vi "DriveModuleReadEncoder.vi"(8 "error in":errorcluster, 11 "ModualNamePrefix":i32) -> (0 "error out":errorcluster, 2 "SWERVE_DRIVE_MODULE_POSITION":T1={"Distance"=0.0, "Angle"={"VALUE"=0.0, "COS"=1.0, "SIN"=0.0}, "P"=FALSE} {"Angle"."SIN" format="%13.4f"; "Angle"."COS" format="%13.4f"; "Angle"."VALUE" format="%13.4f"}, 3 "SWERVE_DRIVE_MODULE_STATE":T3={"Speed"=0.0, "Angle"={"VALUE"=0.0, "COS"=1.0, "SIN"=0.0}} {"Angle"."SIN" format="%13.4f"; "Angle"."COS" format="%13.4f"; "Angle"."VALUE" format="%13.4f"})   [LabVIEW 2023]
uses:
  <vilib>/Rock Robotics/WPI/ThirdParty/JAS_Junk/TrajLib/TypeDef/SWERVE_DRIVE_MODULE_STATE.ctl
  <vilib>/Rock Robotics/WPI/ThirdParty/JAS_Junk/TrajLib/TypeDef/ROTATION2D.ctl
  <vilib>/Rock Robotics/WPI/ThirdParty/JAS_Junk/TrajLib/TypeDef/SWERVE_DRIVE_MODULE_POSITION.ctl
  <vilib>/Rock Robotics/WPI/ThirdParty/JAS_Junk/TrajLib/Conv_Deg_Radians.vi
  <vilib>/Rock Robotics/WPI/ThirdParty/JAS_Junk/TrajLib/Rotation2d_CreateAngle.vi
  DriveGlobal.vi
  <vilib>/Rock Robotics/WPI/ThirdParty/Phoenix6/Phoenix6_Device_RefNumRegistryGet.vi
  <vilib>/Rock Robotics/WPI/MotorControl/WPI_MotorControlRefNum Registry Get.vi
  <vilib>/Rock Robotics/WPI/ThirdParty/REV Robotics/REVLib/SubVI/Public/SPARK Get Encoder Status Velocity.vi
  <vilib>/Rock Robotics/WPI/ThirdParty/REV Robotics/REVLib/SubVI/Public/SPARK Get Encoder Status Position.vi
  <vilib>/Rock Robotics/WPI/ThirdParty/Phoenix6/getters/GetCANcoder_AbsPosition.vi
  <vilib>/Rock Robotics/WPI/ThirdParty/JAS_Junk/TrajLib/Trajectory_Library.lvlib
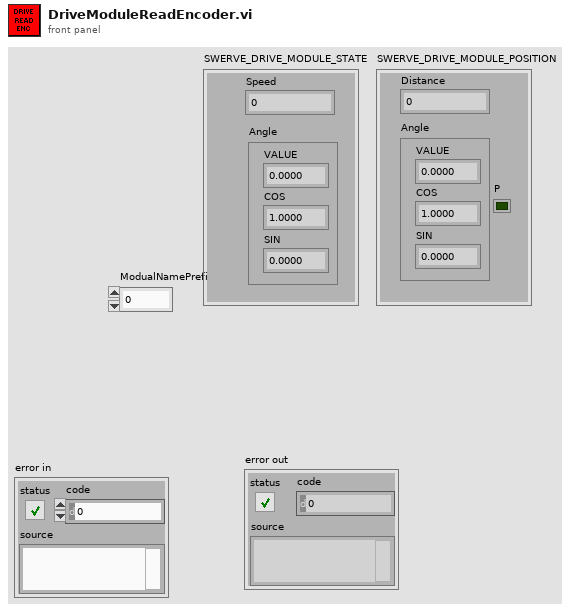
[diagram p1: front panel]
types:
  T1 = typedef "Trajectory_Library.lvlib/SWERVE_DRIVE_MODULE_POSITION.ctl" = cluster{"Distance":dbl, "Angle":T2, "P":bool}
  T2 = typedef "Trajectory_Library.lvlib/ROTATION2D.ctl" = cluster{"VALUE":dbl, "COS":dbl, "SIN":dbl}
  T3 = typedef "Trajectory_Library.lvlib/SWERVE_DRIVE_MODULE_STATE.ctl" = cluster{"Speed":dbl, "Angle":T2}
  T4 = typedef "WPI_MotorControlDeviceRef.ctl" = cluster{"DeviceStatus":errorcluster, "Type":T5, "PWM":cluster{"PWM Channel":T6, "DeadBand":T7}, "CAN":cluster{"Device Number":u8, "SetOutput VI Ref":variant, "GetOutput VI Ref":variant, "Enable VI Ref":variant, "Disable VI Ref":variant, "Data":variant}, "Invert":bool, "DIO PWM":cluster{"PWM \"Enable\" Channel":T6, "DIOChannel":T8, "PWM Rate":dbl}}
  T5 = typedef "WPI_MotorControlType.ctl" = enum16{"PWM", "CAN", "DIO PWM"}
  T6 = typedef "FPGA_DIOPWMChannel.ctl" = enum8{"PWM 0", "PWM 1", "PWM 2", "PWM 3", "PWM 4", "PWM 5", "PWM 6", "PWM 7", "PWM 8", "PWM 9", "PWM MXP 0", "PWM MXP 1", "PWM MXP 2", "PWM MXP 3", "PWM MXP 4", "PWM MXP 5", "PWM MXP 6", "PWM MXP 7", "PWM MXP 8", "PWM MXP 9", "Invalid"}
  T7 = typedef "WPI_PWMDeadband.ctl" = cluster{"Name":string, "maxPositivePwm":i32, "minPositivePwm":i32, "centerPwm":i32, "maxNegativePwm":i32, "minNegativePwm":i32, "angularRange":u16}
  T8 = typedef "FPGA_DIOChannel.ctl" = enum8{"DIO 0", "DIO 1", "DIO 2", "DIO 3", "DIO 4", "DIO 5", "DIO 6", "DIO 7", "DIO 8", "DIO 9", "DIO MXP 0", "DIO MXP 1", "DIO MXP 2", "DIO MXP 3", "DIO MXP 4", "DIO MXP 5", "DIO MXP 6", "DIO MXP 7", "DIO MXP 8", "DIO MXP 9", "DIO MXP 10", "DIO MXP 11", "DIO MXP 12", "DIO MXP 13", "DIO MXP 14", "DIO MXP 15", "SPI Port CS1", "SPI Port CS2", "SPI Port CS3", "SPI Port MISO", "SPI Port MOSI", "Invalid"}
  T9 = typedef "DeviceReference.ctl" = cluster{"CANbus Name":string, "Device Encoding":u32, "Device Name":string}
  T10 = cluster{"Value":dbl, "System Timestamp":dbl, "CANivore Timestamp":dbl, "ECU Timestamp":dbl}
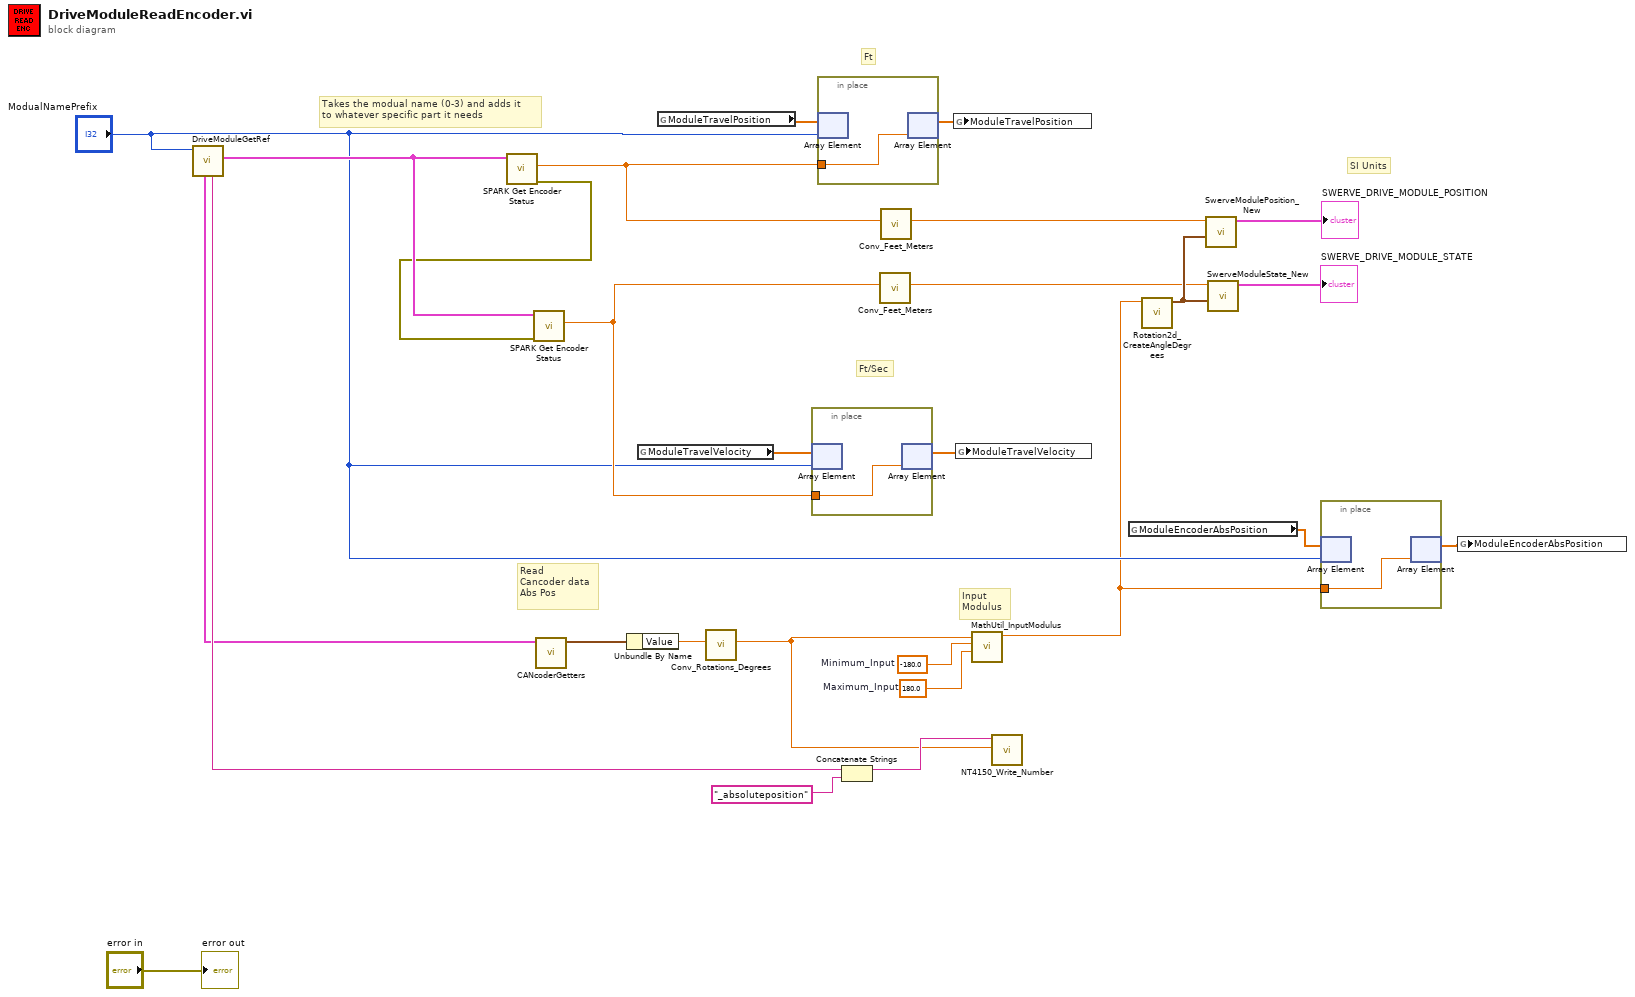
[diagram p0: block diagram]
diagram:
  w21 = -180.0  # Minimum_Input
  w20 = 180.0  # Maximum_Input
  # "SI Units"
  # "Ft/Sec"
  # "Ft"
  # "Read\nCancoder data\nAbs Pos"
  # "Input\nModulus"
  # "Takes the modual name (0-3) and adds it \nto whatever specific part it needs"
  n1 = call "DriveModuleGetRef.vi"("ModualNamePrefix"="ModualNamePrefix") -> ("TravMot"=w16:T4, "EncStr"=w17:string, "SpinAbsAngle"=w14:T9)  [unwired: 5 in, 3 out]
  n2 = call-poly <vilib>:"SPARK Get Encoder Status.vi"("MotorControlDevRef in"=w16) -> ("error out"=w15:errorcluster, "Sensor Position"=w9:dbl)  [unwired: 7 in, 2 out]
  n3 = call-poly <vilib>:"SPARK Get Encoder Status.vi"("error in (no error)"=w15, "MotorControlDevRef in"=w16) -> ("Sensor Velocity"=w5:dbl)  [unwired: 6 in, 3 out]
  n4 = call-poly <vilib>:"CANcoderGetters.vi"("DeviceReference"=w14) -> ("Output"=w13:T10)  [unwired: 9 in, 1 out]
  n5 = Unbundle By Name(w13) -> ("Value"=w12:dbl)
  n6 = global read "DriveGlobal.vi" "ModuleTravelVelocity"() -> (w7:dbl[])
  n7 = global read "DriveGlobal.vi" "ModuleTravelPosition"() -> (w10:dbl[])
  n8 = call <vilib>:"Conv_Rotations_Degrees.vi"("Rotations"=w12) -> ("Degrees"=w11:dbl)  [unwired: 10 in]
  n9 = in-place {
    in-place-border: w5 -> [w28]
    n10 = in-place-array #1(w7, "ModualNamePrefix") -> ()  [unwired: 1 out]
    n11 = in-place-array #1(w28) -> (w6:dbl[])  [unwired: 1 out]
  }
  n12 = in-place {
    in-place-border: w9 -> [w29]
    n13 = in-place-array #2(w10, "ModualNamePrefix") -> ()  [unwired: 1 out]
    n14 = in-place-array #2(w29) -> (w8:dbl[])  [unwired: 1 out]
  }
  n15 = Concatenate Strings(w17, "_absoluteposition" ("refnum name")) -> (w25:string)
  n16 = call <vilib>:"Conv_Feet_Meters.vi"("Feet"=w5) -> ("Meters"=w19:dbl)  [unwired: 10 in]
  n17 = call <vilib>:"Conv_Feet_Meters.vi"("Feet"=w9) -> ("Meters"=w18:dbl)  [unwired: 10 in]
  n18 = global write "DriveGlobal.vi" "ModuleTravelPosition"(w8) -> ()
  n19 = global write "DriveGlobal.vi" "ModuleTravelVelocity"(w6) -> ()
  n20 = call <vilib>:"MathUtil_InputModulus.vi"("Maximum_Input"=w20, "Minimum_Input"=w21, "Input"=w11) -> ("modulus"=w3:dbl)  [unwired: 8 in]
  n21 = call "NT4150_Write_Number.vi"("value"=w11, "name"=w25) -> ()  [unwired: 9 in, 1 out]
  n22 = global read "DriveGlobal.vi" "ModuleEncoderAbsPosition"() -> (w2:dbl[])
  n23 = call <vilib>:"Rotation2d_CreateAngleDegrees.vi"("Angle_Degrees"=w3) -> ("ROTATION"=w24:T2)  [unwired: 10 in]
  n24 = call <vilib>:"SwerveModulePosition_New.vi"("ROTATION"=w24, "Distance"=w18) -> ("SWERVE_DRIVE_MODULE_POSITION"=→"SWERVE_DRIVE_MODULE_POSITION":T1)  [unwired: 9 in]
  n25 = call <vilib>:"SwerveModuleState_New.vi"("ROTATION"=w24, "Speed"=w19) -> ("SWERVE_DRIVE_MODULE_STATE"=→"SWERVE_DRIVE_MODULE_STATE":T3)  [unwired: 9 in]
  n26 = in-place {
    in-place-border: w3 -> [w30]
    n27 = in-place-array #3(w2, "ModualNamePrefix") -> ()  [unwired: 1 out]
    n28 = in-place-array #3(w30) -> (w1:dbl[])  [unwired: 1 out]
  }
  n29 = global write "DriveGlobal.vi" "ModuleEncoderAbsPosition"(w1) -> ()
  "error out" <- "error in"
